vi "USB.vi"() -> ()   [LabVIEW 2019]
panel:
  in  "Stop":bool
  out "read buffer":string
  out "error out":errorcluster
  out "Interface Description":string
  in  "VISA resource name":refnum<visa-resource-name>
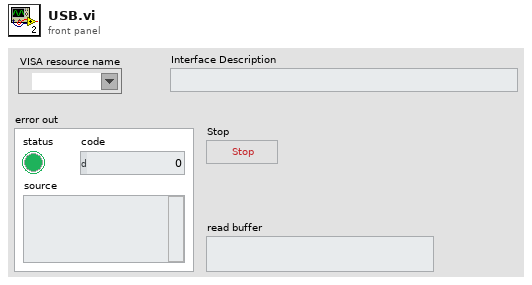
[diagram p1: front panel]
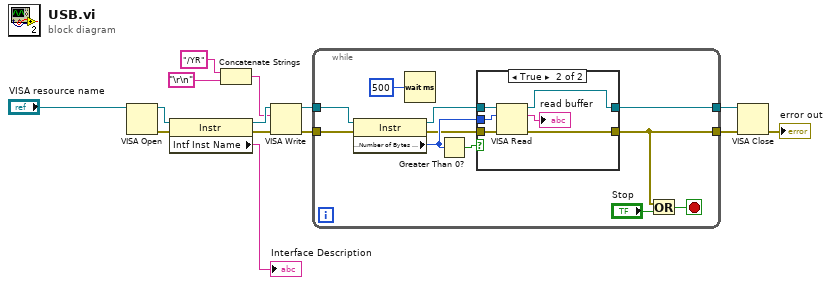
[diagram p0: block diagram]
diagram:
  n1 = VISA Open(VISA resource name="VISA resource name") -> (VISA resource name=w14:refnum<visa-resource-name>, error out=w12:errorcluster)  [unwired: 4 in]
  n2 = property class="Instr"(reference=w14, error in=w12) -> (reference out=w9:refnum<visa-resource-name>, error out=w11:errorcluster, "Intf Inst Name"=→"Interface Description":string)
  n3 = Concatenate Strings("/YR" ("write buffer"), "\r\n") -> (w4:string)
  n4 = VISA Write(VISA resource name=w9, write buffer=w4, error in (no error)=w11) -> (VISA resource name out=w7:refnum<visa-resource-name>, error out=w8:errorcluster)  [unwired: 1 out]
  n5 = while {
    tunnel: w7 -> [w20]
    tunnel: w8 -> [w19]
    tunnel: [w18] -> w2
    tunnel: [w15] -> w1
    stop <- w16 stop-if-true
    n6 = property class="Instr"(reference=w20, error in=w19) -> (reference out=w21:refnum<visa-resource-name>, error out=w22:errorcluster, "Serial Settings:Number of Bytes at Serial Port"=w24:u32)
    n7 = Wait (ms)(milliseconds to wait=u32 500) -> ()  [unwired: 1 out]
    n8 = Greater Than 0?(x=w24) -> (x > 0?=w23:bool)
    n9 = case shown="True" w23 {
      tunnel: w21 -> [w27 w33]
      tunnel: [w27 w32] -> w18
      tunnel: w22 -> [w26 w31]
      tunnel: [w26 w30] -> w15
      tunnel: w24 -> [_ w29]
      frame False {
      }
      frame True {
        n10 = VISA Read(VISA resource name=w33, byte count=w29, error in (no error)=w31) -> (VISA resource name out=w32:refnum<visa-resource-name>, read buffer=→"read buffer":string, error out=w30:errorcluster)  [unwired: 1 out]
      }
    }
    n11 = Or(x=w15, y="Stop") -> (x .or. y?=w16:bool)
  }
  n12 = VISA Close(VISA resource name=w2, error in (no error)=w1) -> (error out=→"error out":errorcluster)
